vi "Settings Path - Default--Const.vi"() -> (2 "Default Settings Path":path)   [LabVIEW 2017, in "DTacq Plot Display Library.lvlib"]
doc: "Full name and path to the default settings ini file"
uses:
  DTacq Plot Display Library.lvlib
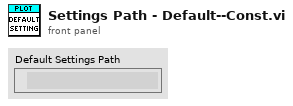
[diagram p1: front panel]
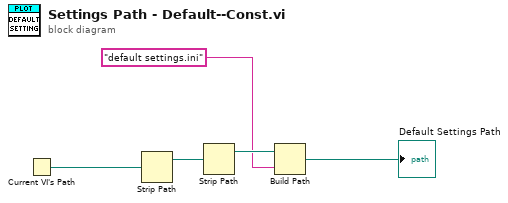
[diagram p0: block diagram]
diagram:
  n1 = Current VI's Path() -> (path=w5:path)
  n2 = Strip Path(path=w5) -> (stripped path=w4:path)  [unwired: 1 out]
  n3 = Strip Path(path=w4) -> (stripped path=w3:path)  [unwired: 1 out]
  n4 = Build Path(base path=w3, name or relative path="default settings.ini") -> (appended path=→"Default Settings Path":path)
